vi "Read Identity Toolkit URL.vi"(8 "error in (no error)":errorcluster, 11 "firebase in":refnum<class "firebase.lvclass">) -> (0 "error out":errorcluster, 2 "Identity Toolkit URL":string, 3 "firebase out":refnum<class "firebase.lvclass">)   [LabVIEW 2019, in "firebase.lvclass"]
uses:
  firebase.lvclass
  firebase.lvclass/firebase.ctl
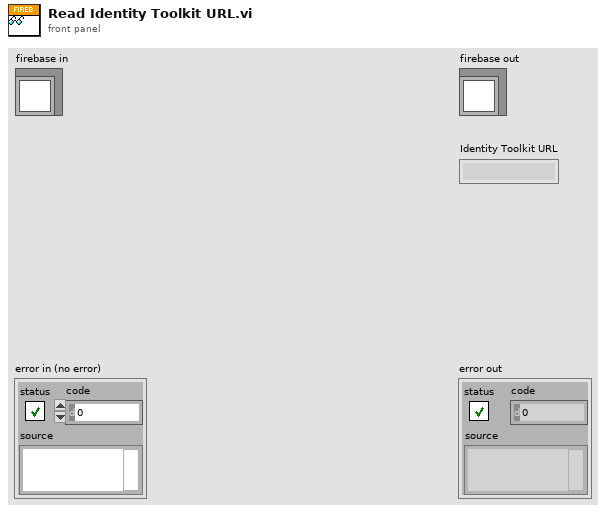
[diagram p1: front panel]
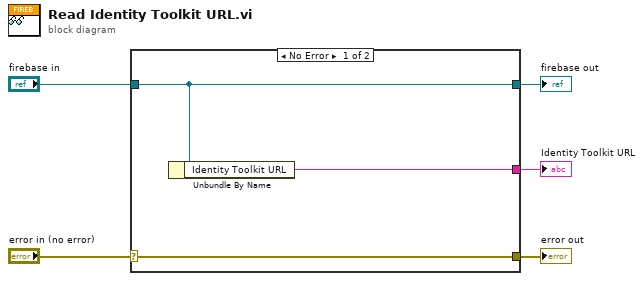
[diagram p0: block diagram]
diagram:
  n1 = case shown="No Error" "error in (no error)" {
    selector: "error in (no error)" -> [w8 w9]
    tunnel: [w8 w9] -> w4
    tunnel: [w7 w10] -> w2
    tunnel: "firebase in" -> [w7 w10]
    tunnel: [w6 _] -> w1
    frame No Error {
      n2 = Unbundle By Name(w7) -> ("Identity Toolkit URL"=w6:string)
    }
    frame Error {
    }
  }
  "error out" <- w4
  "firebase out" <- w2
  "Identity Toolkit URL" <- w1
